vi "电信181原源.VI"() -> ()   [LabVIEW 2020]
uses:
  <vilib>/Utility/file.llb/Read Delimited Spreadsheet (DBL).vi
  <vilib>/Utility/file.llb/Write Delimited Spreadsheet (DBL).vi
panel:
  out "坐标显示":string
  out "电容电压":dbl
  in  "选项卡控件":enum32{"电容充放电波形采集", "充电波形 ", "放电波形"}(tab)
  out "电容充放电波形采集":dbl(graph)
  out "充电波形":dbl[](graph)
  out "放电波形":dbl[](graph)
  out "充放电状态显示":bool
  in  "退出":bool
  in  "回放":bool
  in  "保存":bool
  in  "开始":bool
  out "放电时间 (s)":dbl=5.0
  out "充电时间 (s)":dbl=5.0
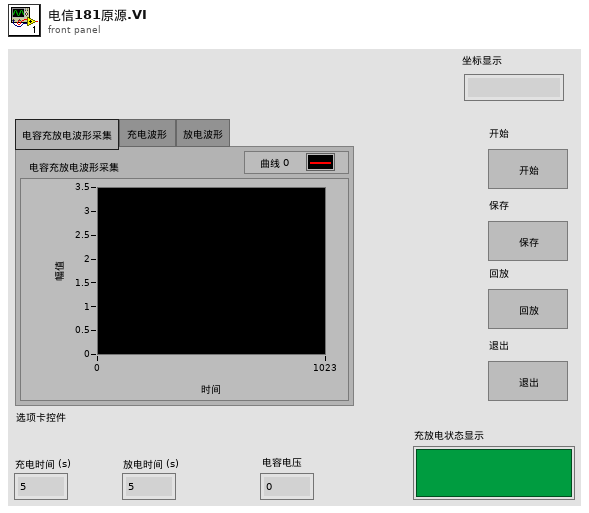
[diagram p1: front panel]
types:
  T1 = typedef "LVPoint32TypeDef.ctl" = cluster{"Horizontal":i32, "Vertical":i32}
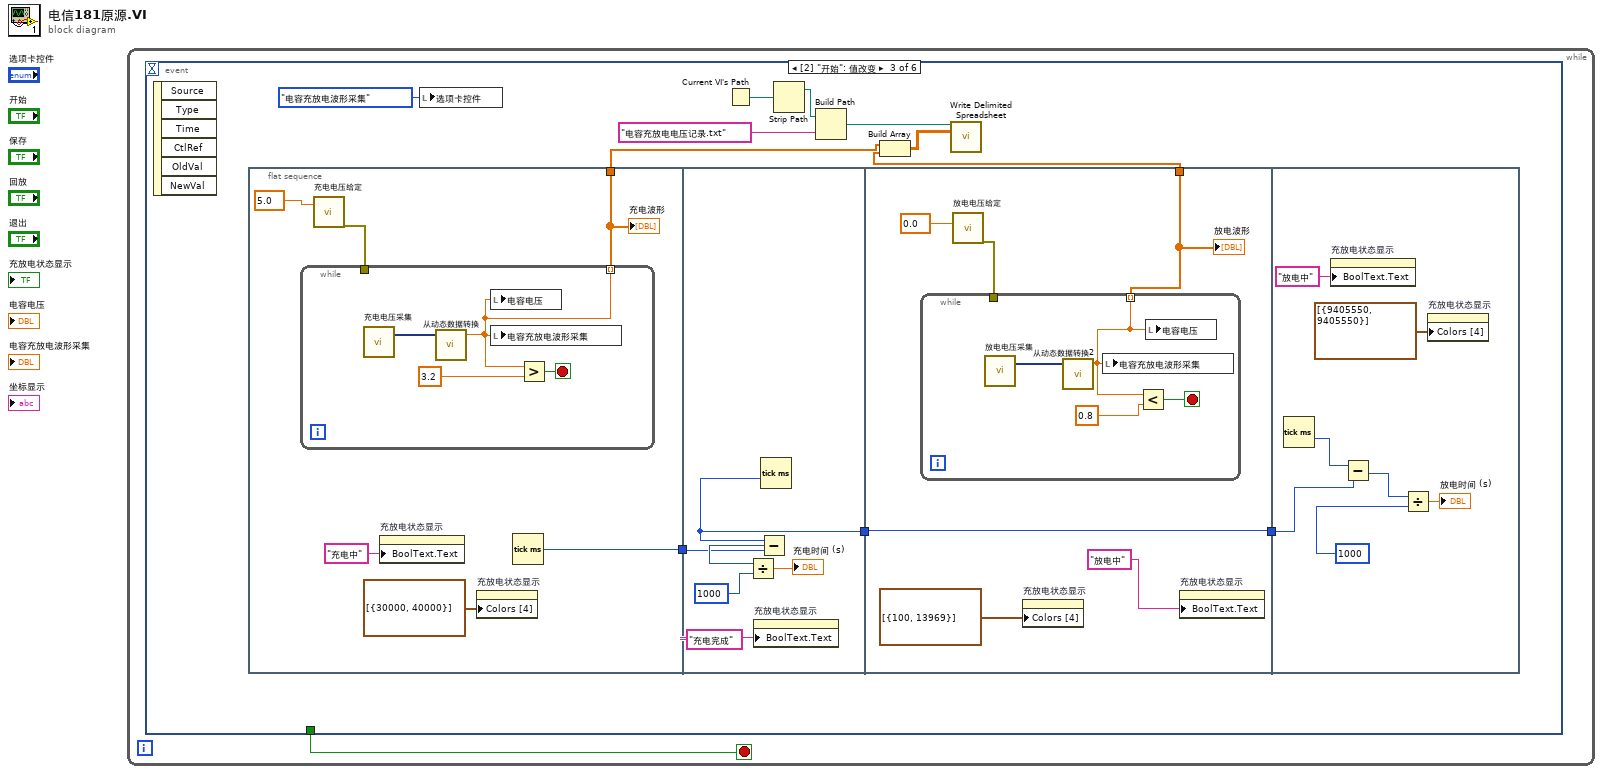
[diagram p0: block diagram]
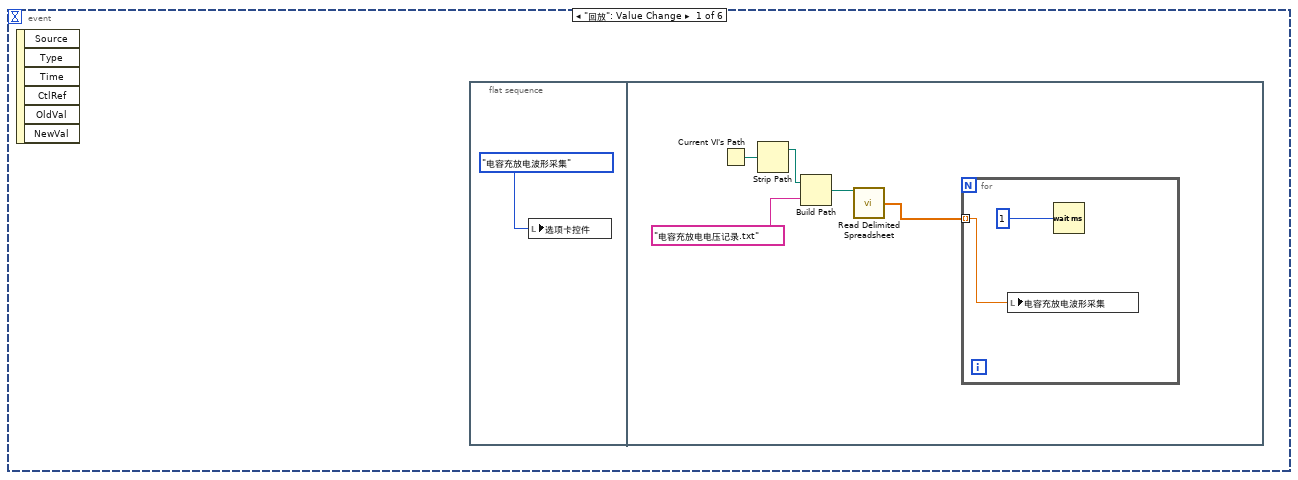
[diagram p2: hidden frame]
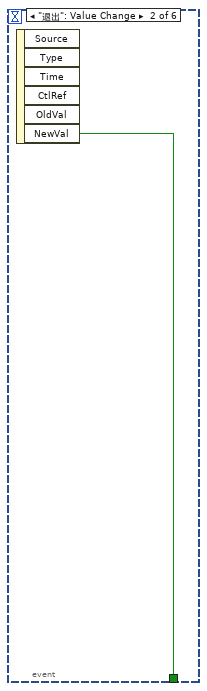
[diagram p3: hidden frame]
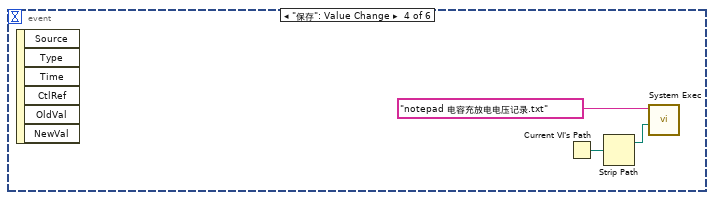
[diagram p4: hidden frame]
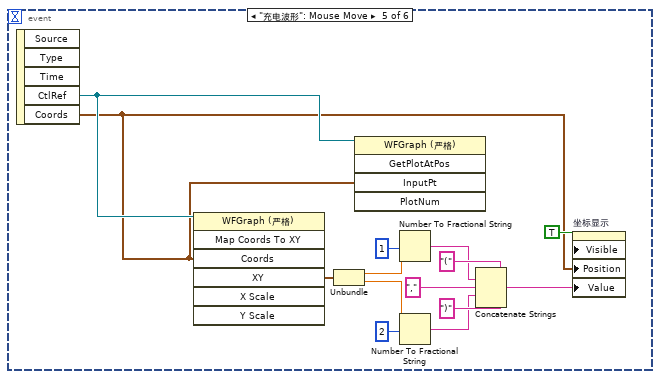
[diagram p5: hidden frame]
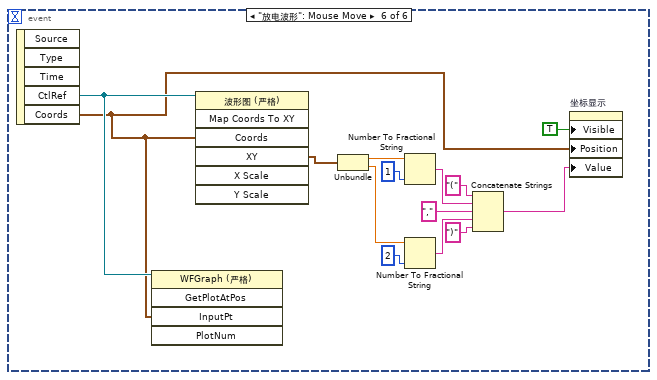
[diagram p6: hidden frame]
diagram:
  n1 = while {
    stop <- w1 stop-if-true
    n2 = event shown="[2] \"开始\": 值改变" {
      selector: _ -> [_ _ _ _ _ _]
      dyn-events: _ -> [_ _ _ _ _ _]
      timeout: _ -> [_ _ _ _ _ _]
      tunnel: [_ w10 _ _ _ _] -> w1
      event "回放": Value Change {
        n3 = event-data() -> ()  [unwired: 1 in, 6 out]
        n4 = flat-sequence {
          frame #0 {
            n5 = local write "选项卡控件"(enum32{"电容充放电波形采集", "充电波形 ", "放电波形"}."电容充放电波形采集" ("选项卡控件")) -> ()
          }
          frame #1 {
            n6 = Current VI's Path() -> (path=w7:path)
            n7 = Strip Path(path=w7) -> (stripped path=w6:path)  [unwired: 1 out]
            n8 = Build Path(base path=w6, name or relative path="电容充放电电压记录.txt") -> (appended path=w4:path)
            n9 = call-poly <vilib>:"Read Delimited Spreadsheet.vi"("file path (dialog if empty)"=w4) -> ("first row"=w3:dbl[])  [unwired: 9 in, 5 out]
            n10 = for {
              tunnel: w3 -> [w8] mode=indexing
              n11 = local write "电容充放电波形采集"(w8) -> ()
              n12 = Wait (ms)(milliseconds to wait=u32 1 ("等待时间（毫秒）")) -> ()  [unwired: 1 out]
            }
          }
        }
      }
      event "退出": Value Change {
        n13 = event-data() -> ("NewVal"=w10:bool)  [unwired: 1 in, 5 out]
      }
      event "开始": Value Change {
        n14 = event-data() -> ()  [unwired: 1 in, 6 out]
        n15 = flat-sequence {
          tunnel: [w24] -> w17
          tunnel: [w27] -> w15
          tunnel: [w33] -> w16
          tunnel: w15 -> [w36]
          tunnel: w16 -> [w41]
          tunnel: [w41] -> w14
          tunnel: [w38] -> w12
          tunnel: w14 -> [w48]
          frame #0 {
            n16 = call "充电电压给定"("data"=5.0 ("timeout (s)")) -> ("error out"=w22:errorcluster)  [unwired: 17 in, 1 out]
            n17 = while {
              tunnel: [w29] -> w24 mode=indexing
              tunnel: w22 -> [_]
              stop <- w31 stop-if-true
              n18 = call "充电电压采集"() -> ("data"=w28:dynamicdata)  [unwired: 17 in, 2 out]
              n19 = call "从动态数据转换"("Dynamic Data Type"=w28) -> ("Scalar"=w29:dbl)  [unwired: 3 in]
              n20 = local write "电容电压"(w29) -> ()
              n21 = local write "电容充放电波形采集"(w29) -> ()
              n22 = Greater?(x=w29, y=3.2) -> (0:w31:bool)
            }
            "充电波形" <- w24
            n23 = property on="充放电状态显示" class="Bool (严格)"("BoolText.Text"="充电中") -> ()  [unwired: 2 in, 2 out]
            n24 = property on="充放电状态显示" class="Bool (严格)"("Colors [4]"=cluster{i32, i32}[] [{30000, 40000}]) -> ()  [unwired: 2 in, 2 out]
            n25 = Tick Count (ms)() -> (millisecond timer value=w27:u32)
          }
          frame #1 {
            n26 = property on="充放电状态显示" class="Bool (严格)"("BoolText.Text"="充电完成") -> ()  [unwired: 2 in, 2 out]
            n27 = Tick Count (ms)() -> (millisecond timer value=w33:u32)
            n28 = Subtract(x=w33, y=w36) -> (x-y=w37:u32)
            n29 = Divide(x=w37, y=u32 1000) -> (x/y=→"充电时间 (s)":dbl)
          }
          frame #2 {
            n30 = call "放电电压给定"("data"=0.0 ("timeout (s)")) -> ("error out"=w39:errorcluster)  [unwired: 17 in, 1 out]
            n31 = while {
              tunnel: [w45] -> w38 mode=indexing
              tunnel: w39 -> [_]
              stop <- w47 stop-if-true
              n32 = call "放电电压采集"() -> ("data"=w44:dynamicdata)  [unwired: 17 in, 2 out]
              n33 = call "从动态数据转换2"("Dynamic Data Type"=w44) -> ("Scalar"=w45:dbl)  [unwired: 3 in]
              n34 = local write "电容充放电波形采集"(w45) -> ()
              n35 = Less?(x=w45, y=0.8) -> (x < y?=w47:bool)
              n36 = local write "电容电压"(w45) -> ()
            }
            "放电波形" <- w38
            n37 = property on="充放电状态显示" class="Bool (严格)"("Colors [4]"=cluster{i32, i32}[] [{100, 13969}]) -> ()  [unwired: 2 in, 2 out]
            n38 = property on="充放电状态显示" class="Bool (严格)"("BoolText.Text"="放电中") -> ()  [unwired: 2 in, 2 out]
          }
          frame #3 {
            n39 = Tick Count (ms)() -> (millisecond timer value=w52:u32)
            n40 = property on="充放电状态显示" class="Bool (严格)"("BoolText.Text"="放电中") -> ()  [unwired: 2 in, 2 out]
            n41 = Subtract(x=w52, y=w48) -> (x-y=w54:u32)
            n42 = Divide(x=w54, y=u32 1000) -> (x/y=→"放电时间 (s)":dbl)
            n43 = property on="充放电状态显示" class="Bool (严格)"("Colors [4]"=cluster{i32, i32}[] [{9405550, 9405550}]) -> ()  [unwired: 2 in, 2 out]
          }
        }
        n44 = local write "选项卡控件"(enum32{"电容充放电波形采集", "充电波形 ", "放电波形"}."电容充放电波形采集" ("选项卡控件")) -> ()
        n45 = Current VI's Path() -> (path=w19:path)
        n46 = Strip Path(path=w19) -> (stripped path=w21:path)  [unwired: 1 out]
        n47 = Build Path(base path=w21, name or relative path="电容充放电电压记录.txt") -> (appended path=w18:path)
        n48 = Build Array(w17, w12) -> (w11:dbl[][])
        n49 = call-poly <vilib>:"Write Delimited Spreadsheet.vi"("file path (dialog if empty)"=w18, "2D data"=w11) -> ()  [unwired: 12 in, 2 out]
      }
      event "保存": Value Change {
        n50 = event-data() -> ()  [unwired: 1 in, 6 out]
        n51 = Current VI's Path() -> (path=w57:path)
        n52 = Strip Path(path=w57) -> (stripped path=w55:path)  [unwired: 1 out]
        n53 = call <vilib>:"System Exec.vi"("working directory"=w55, "command line"="notepad 电容充放电电压记录.txt") -> ()  [unwired: 6 in, 4 out]
      }
      event "充电波形": Mouse Move {
        n54 = event-data() -> ("CtlRef"=w59:refnum<vi>, "Coords"=w58:T1)  [unwired: 1 in, 3 out]
        n55 = invoke class="WFGraph (严格)" method="Map Coords To XY"(reference=w59, "Coords"=w58) -> ("XY"=w62:cluster{"X":dbl, "Y":dbl})  [unwired: 5 in, 6 out]
        n56 = Unbundle(w62) -> ("X"=w61:dbl, "Y"=w60:dbl)
        n57 = invoke class="WFGraph (严格)" method="GetPlotAtPos"(reference=w59, "InputPt"=w58) -> ()  [unwired: 3 in, 5 out]
        n58 = Number To Fractional String(number=w61, precision (6)=i16 1 ("精度(6)")) -> (F-format string=w66:string)  [unwired: 2 in]
        n59 = Number To Fractional String(number=w60, precision (6)=i16 2 ("精度(6)")) -> (F-format string=w65:string)  [unwired: 2 in]
        n60 = Concatenate Strings("(", w66, ",", w65, ")") -> (w64:string)
        n61 = property on="坐标显示" class="Str"("Visible"=TRUE ("可见"), "Position"=w58, "Value"=w64) -> ()  [unwired: 2 in, 2 out]
      }
      event "放电波形": Mouse Move {
        n62 = event-data() -> ("CtlRef"=w73:refnum<vi>, "Coords"=w72:T1)  [unwired: 1 in, 3 out]
        n63 = invoke class="WFGraph (严格)" method="GetPlotAtPos"(reference=w73, "InputPt"=w72) -> ()  [unwired: 3 in, 5 out]
        n64 = invoke class="波形图 (严格)" method="Map Coords To XY"(reference=w73, "Coords"=w72) -> ("XY"=w74:cluster{"X":dbl, "Y":dbl})  [unwired: 5 in, 6 out]
        n65 = Unbundle(w74) -> ("X"=w85:dbl, "Y"=w83:dbl)
        n66 = Number To Fractional String(number=w85, precision (6)=i16 1 ("精度(6)")) -> (F-format string=w78:string)  [unwired: 2 in]
        n67 = Number To Fractional String(number=w83, precision (6)=i16 2 ("精度(6)")) -> (F-format string=w77:string)  [unwired: 2 in]
        n68 = Concatenate Strings("(", w78, ",", w77, ")") -> (w75:string)
        n69 = property on="坐标显示" class="Str"("Visible"=TRUE ("可见"), "Position"=w72, "Value"=w75) -> ()  [unwired: 2 in, 2 out]
      }
    }
  }
